vi "Handle.vi"(11 "TEMPLATE Queue in":refnum<class "TEMPLATE Queue.lvclass">) -> (2 "Destroy?":bool, 3 "TEMPLATE Queue out":refnum<class "TEMPLATE Queue.lvclass">)   [LabVIEW 2021, in "_Template.lvlib" / "Templates.lvlib" / "TEM Queue.lvlib" / "TEMPLATE Queue.lvclass"]
uses:
  TEMPLATE Queue.lvclass
  TEMPLATE Queue.lvclass/TEMPLATE Queue.ctl
  <vilib>/Nathan Davis/jettl/jettl/Queue/Queue.lvclass
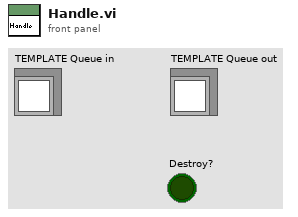
[diagram p1: front panel]
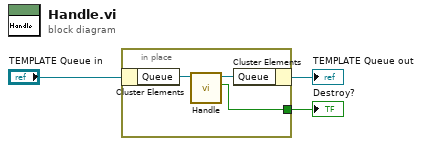
[diagram p0: block diagram]
diagram:
  n1 = in-place {
    in-place-border: [w4] -> w1
    n2 = in-place-cluster #1("TEMPLATE Queue in") -> ("Queue"=w6:refnum<class "Queue.lvclass">)
    n3 = call-dynamic "Handle.vi"("jettl in"=w6) -> ("Destroy?"=w4:bool, "jettl out"=w5:refnum<class "Queue.lvclass">)  [unwired: 9 in]
    n4 = in-place-cluster #1("Queue"=w5) -> (→"TEMPLATE Queue out":refnum<class "TEMPLATE Queue.lvclass">)
  }
  "Destroy?" <- w1
